vi "SPD.HV_Bias SubTest.vi"(0 "SPD.Stand Ctrl in":T4={"spdDeviceSession"={"spdRef"=0, "connected"=FALSE, "spdName"="", "specification"={"diod case"=enum."default", "type"=enum."Unknown", "frequency"=enum."Unknown"}, "hidSPD.Controller"={"TSet"=0.0, "HV_bias"=0.0, "DDS_stb_code"=0}, "hidSPD.Sturtup Values"={"TSet"=0.0, "HV_bias"=0.0, "DDS_stb_code"=0}}, "DevBSession"={"DevBRef"="", "connected"=FALSE}, "FreqCSession"={"FreqCRef"="", "timeout"=0.0, "Gate"=0.0, "connected"=FALSE}, "8164BSession"={"Connection ID"=refnum, "Connected"=FALSE, "Info"="", "Slots Info"=[]}, "LeCroySession"={"LeCroySession"="", "connected"=FALSE}, "Events"={"DCRTest"=refnum, "Stop"=refnum}, "configFile"={"configFile ref"=refnum, "configFile path"=path "", "equipmentFile ref"=refnum}, "SPD.Meas Grid"={"DateTime"="", "DT"=[], "Insensitivity"=[], "Temprature"=[], "Stb_code"=[], "HV_Bias"=[]}, "SPD.Queues"={"state queue"=refnum}, "Console"=refnum} {"spdDeviceSession"."hidSPD.Sturtup Values"."HV_bias" format="%#_6p, V"; "spdDeviceSession"."hidSPD.Sturtup Values"."TSet" format="%#_6p, DegC"; "spdDeviceSession"."hidSPD.Controller"."HV_bias" format="%#_6p, V"; "spdDeviceSession"."hidSPD.Controller"."TSet" format="%#_6p, DegC"}, 5 "SPD.HV_bias Test Limits":T1, 11 "Error In":errorcluster, 12 "Progress":refnum<vi>, 13 "Graph":refnum<vi>) -> (4 "SPD.Stand Ctrl out":T4={"spdDeviceSession"={"spdRef"=0, "connected"=FALSE, "spdName"="", "specification"={"diod case"=enum."default", "type"=enum."Unknown", "frequency"=enum."Unknown"}, "hidSPD.Controller"={"TSet"=0.0, "HV_bias"=0.0, "DDS_stb_code"=0}, "hidSPD.Sturtup Values"={"TSet"=0.0, "HV_bias"=0.0, "DDS_stb_code"=0}}, "DevBSession"={"DevBRef"="", "connected"=FALSE}, "FreqCSession"={"FreqCRef"="", "timeout"=0.0, "Gate"=0.0, "connected"=FALSE}, "8164BSession"={"Connection ID"=refnum, "Connected"=FALSE, "Info"="", "Slots Info"=[]}, "LeCroySession"={"LeCroySession"="", "connected"=FALSE}, "Events"={"DCRTest"=refnum, "Stop"=refnum}, "configFile"={"configFile ref"=refnum, "configFile path"=path "", "equipmentFile ref"=refnum}, "SPD.Meas Grid"={"DateTime"="", "DT"=[], "Insensitivity"=[], "Temprature"=[], "Stb_code"=[], "HV_Bias"=[]}, "SPD.Queues"={"state queue"=refnum}, "Console"=refnum} {"spdDeviceSession"."hidSPD.Sturtup Values"."HV_bias" format="%#_6p, V"; "spdDeviceSession"."hidSPD.Sturtup Values"."TSet" format="%#_6p, DegC"; "spdDeviceSession"."hidSPD.Controller"."HV_bias" format="%#_6p, V"; "spdDeviceSession"."hidSPD.Controller"."TSet" format="%#_6p, DegC"}, 6 "last HV_bias":dbl, 8 "Clicks Count":dbl, 10 "result":bool, 15 "Error Out":errorcluster)   [LabVIEW 2018]
uses:
  typedefs/SPD.Stand Ctrl.ctl
  Instruments/SPD HID Interface/hidSPDLibForLabView/LibVIs/hidSPD Controls/hidSPD Device Session.ctl
  Instruments/SPD HID Interface/hidSPDLibForLabView/LibVIs/hidSPD Controls/hidSPD.SPD specification.ctl
  Instruments/SPD HID Interface/hidSPDLibForLabView/LibVIs/hidSPD Controls/hidSPD SPD Diod Case.ctl
  Instruments/SPD HID Interface/hidSPDLibForLabView/LibVIs/hidSPD Controls/hidSPD SPD Type.ctl
  Instruments/SPD HID Interface/hidSPDLibForLabView/LibVIs/hidSPD Controls/hidSPD.STB Frequency.ctl
  Instruments/SPD HID Interface/hidSPDLibForLabView/LibVIs/hidSPD Controls/hidSPD Controller.ctl
  Instruments/KC705 DevBoard/typedefs/DevB.Session.ctl
  Instruments/KeySight 53230A/typedefs/FreqC.Session.ctl
  Instruments/KeySight 8164B/KeySight 8164B LAN InstrLib/typedefs/KeySight 8164B control.ctl
  Instruments/LeCroy SDA830/typedefs/LeCroy.Session.ctl
  typedefs/SPD.Events.ctl
  ConfigFile/SPD.Config File ctrl.ctl
  <vilib>/Utility/config.llb/Config Data RefNum.ctl
  typedefs/SPD.Meas Grid.ctl
  typedefs/SPD.Queues.ctl
  typedefs/SPD.Stand state.ctl
  SPD.HV_Bias Test Limits.vi
  SubVIs/Min_Max.ctl
  SubVIs/comparison mode.ctl
  Instruments/SPD HID Interface/hidSPDLibForLabView/LibVIs/hidSPD Controls/hidSPD Controller Setup Report.ctl
  <vilib>/Analysis/1siggen.llb/Ramp Pattern by Delta.vi
  Instruments/SPD HID Interface/hidSPDLibForLabView/LibVIs/hidSPD Write Report/hidSPD Setup Controller.vi
  Instruments/SPD HID Interface/hidSPDLibForLabView/hidSPDLibForLabView.lvlib
  <vilib>/Analysis/NI_AALBase.lvlib
  Instruments/KeySight 8164B/KeySight 8164B LAN InstrLib.lvlib
  <vilib>/Utility/config.llb/NI_LVConfig.lvlib
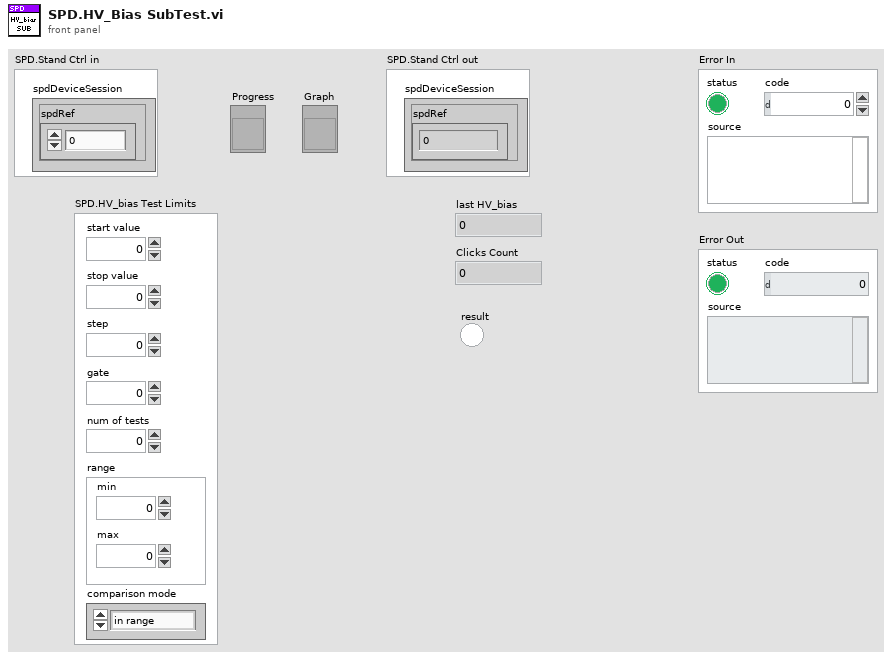
[diagram p1: front panel]
types:
  T1 = typedef "SPD.HV_Bias Test Limits.vi" = cluster{"start value":dbl, "stop value":dbl, "step":dbl, "gate":dbl, "num of tests":dbl, "range":T2, "comparison mode":T3}
  T2 = typedef "Min_Max.ctl" = cluster{"min":dbl, "max":dbl}
  T3 = typedef "comparison mode.ctl" = enum16{"in range", "bigger then min", "bigger then max", "less then min", "less then max"}
  T4 = typedef "SPD.Stand Ctrl.ctl" = cluster{"spdDeviceSession":T5, "DevBSession":T11, "FreqCSession":T12, "8164BSession":T13, "LeCroySession":T14, "Events":T15, "configFile":T16, "SPD.Meas Grid":T18, "SPD.Queues":T19, "Console":refnum<vi>}
  T5 = typedef "hidSPDLibForLabView.lvlib/hidSPD Device Session.ctl" = cluster{"spdRef":u64, "connected":bool, "spdName":string, "specification":T6, "hidSPD.Controller":T10, "hidSPD.Sturtup Values":T10}
  T6 = typedef "hidSPDLibForLabView.lvlib/hidSPD.SPD specification.ctl" = cluster{"diod case":T7, "type":T8, "frequency":T9}
  T7 = typedef "hidSPDLibForLabView.lvlib/hidSPD SPD Diod Case.ctl" = enum16{"Unknown", "default", "butterfly"}
  T8 = typedef "hidSPDLibForLabView.lvlib/hidSPD SPD Type.ctl" = enum16{"Unknown", "Free Run", "Gate"}
  T9 = typedef "hidSPDLibForLabView.lvlib/hidSPD.STB Frequency.ctl" = enum16{"Unknown", "312", "1250"}
  T10 = typedef "hidSPDLibForLabView.lvlib/hidSPD Controller.ctl" = cluster{"TSet":sgl, "HV_bias":sgl, "DDS_stb_code":u16}
  T11 = typedef "DevB.Session.ctl" = cluster{"DevBRef":refnum<visa-resource-name>, "connected":bool}
  T12 = typedef "FreqC.Session.ctl" = cluster{"FreqCRef":refnum<visa-resource-name>, "timeout":dbl, "Gate":dbl, "connected":bool}
  T13 = typedef "KeySight 8164B LAN InstrLib.lvlib/KeySight 8164B control.ctl" = cluster{"Connection ID":refnum<k5>, "Connected":bool, "Info":string, "Slots Info":string[]}
  T14 = typedef "LeCroy.Session.ctl" = cluster{"LeCroySession":refnum<visa-resource-name>, "connected":bool}
  T15 = typedef "SPD.Events.ctl" = cluster{"DCRTest":refnum<user-event>, "Stop":refnum<user-event>}
  T16 = typedef "SPD.Config File ctrl.ctl" = cluster{"configFile ref":T17, "configFile path":path, "equipmentFile ref":T17}
  T17 = typedef "NI_LVConfig.lvlib/Config Data RefNum.ctl" = refnum<k1>
  T18 = typedef "SPD.Meas Grid.ctl" = cluster{"DateTime":string, "DT":dbl[], "Insensitivity":dbl[], "Temprature":dbl[], "Stb_code":dbl[], "HV_Bias":dbl[][][][]}
  T19 = typedef "SPD.Queues.ctl" = cluster{"state queue":refnum<queue>}
  T20 = typedef "hidSPDLibForLabView.lvlib/hidSPD Controller Setup Report.ctl" = cluster{"TSet":sgl, "HV_bias":sgl, "DDS_stb_code":u16, "SPD_reset":u16, "MCU_reset":u16}
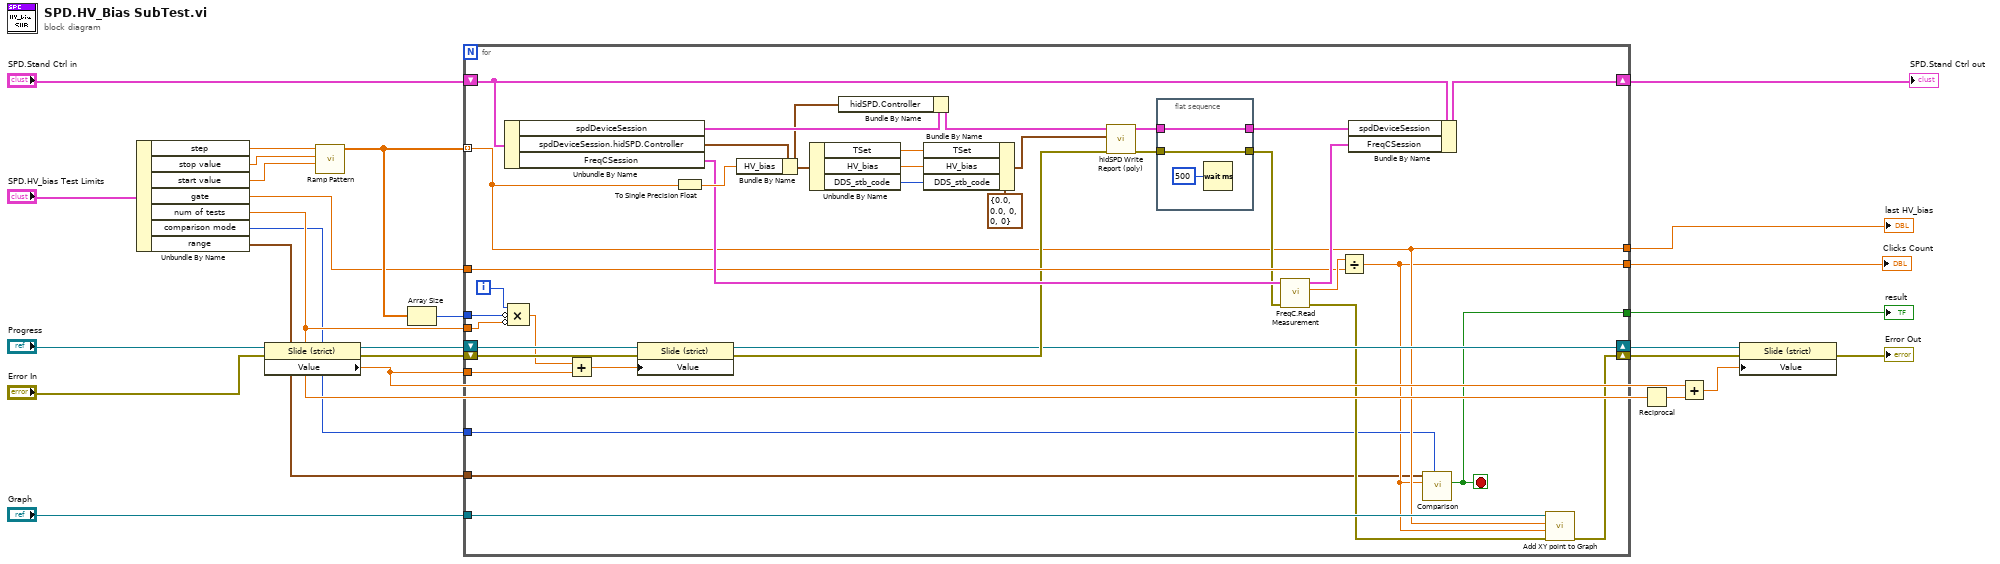
[diagram p0: block diagram]
diagram:
  n1 = Unbundle By Name("SPD.HV_bias Test Limits") -> ("step"=w7:dbl, "stop value"=w6:dbl, "start value"=w5:dbl, "gate"=w4:dbl, "num of tests"=w3:dbl, "comparison mode"=w2:T3, "range"=w1:T2)
  n2 = property class="Slide (strict)"(reference="Progress", error in="Error In") -> (reference out=w21:refnum<vi>, error out=w19:errorcluster, "Value"=w12:dbl)
  n3 = call-poly <vilib>:"Ramp Pattern.vi"("start"=w5, "end"=w6, "delta"=w7) -> ("Ramp Pattern"=w9:dbl[])  [unwired: 6 in, 2 out]
  n4 = Array Size(array=w9) -> (size(s)=w24:i32)
  n5 = for {
    shift-right: [w36] -> w14
    shift-left: w19 -> [w43]
    shift-right: [w53] -> w25
    shift-left: "SPD.Stand Ctrl in" -> [w57]
    tunnel: w9 -> [w38] mode=indexing
    tunnel: w4 -> [w49]
    tunnel: [w35] -> w18
    tunnel: [w38] -> w16
    tunnel: w24 -> [w44]
    shift-right: [w41] -> w15
    shift-left: w21 -> [w40]
    tunnel: "Graph" -> [w39]
    tunnel: [w33] -> w17
    tunnel: w2 -> [w34]
    tunnel: w12 -> [w28]
    tunnel: w1 -> [w31]
    tunnel: w3 -> [w30]
    i -> [w32]
    stop <- w35 stop-if-true
    n6 = Unbundle By Name(w57) -> ("spdDeviceSession"=w64:T5, "spdDeviceSession.hidSPD.Controller"=w62:T10, "FreqCSession"=w51:T12)
    n7 = Compound Arithmetic op=MULTIPLY(w32, invert w44, invert w30) -> (w29:dbl)
    n8 = Add(x=w29, y=w28) -> (x+y=w27:dbl)
    n9 = property class="Slide (strict)"(reference=w40, error in=w43, "Value"=w27) -> (reference out=w41:refnum<vi>, error out=w42:errorcluster)
    n10 = To Single Precision Float(number=w38) -> (single precision float=w52:sgl)
    n11 = Bundle By Name(cluster=w62, "HV_bias"=w52) -> (w55:T10)
    n12 = Unbundle By Name(w55) -> ("TSet"=w61:sgl, "HV_bias"=w60:sgl, "DDS_stb_code"=w59:u16)
    n13 = Bundle By Name(cluster=w64, "hidSPD.Controller"=w55) -> (w56:T5)
    n14 = Bundle By Name(cluster=T20 {"TSet"=0.0, "HV_bias"=0.0, "DDS_stb_code"=0, "SPD_reset"=0, "MCU_reset"=0} ("hidSPD Controller Setup report"), "TSet"=w61, "HV_bias"=w60, "DDS_stb_code"=w59) -> (w58:T20)
    n15 = call-poly "hidSPD Write Report (poly).vi"("error in (no error)"=w42, "hidSPD Controller Setup report"=w58, "spdDevSession in"=w56) -> ("error out"=w47:errorcluster, "spdDevSession out"=w48:T5)  [unwired: 7 in]
    n16 = flat-sequence {
      tunnel: [w67] -> w45
      tunnel: w48 -> [w67]
      tunnel: [w66] -> w46
      tunnel: w47 -> [w66]
      frame #0 {
        n17 = Wait (ms)(milliseconds to wait=u32 500) -> ()  [unwired: 1 out]
      }
    }
    n18 = call "FreqC.Read Measurement.vi"("error In"=w46, "FreqC Session in"=w51) -> ("error out"=w37:errorcluster, "Measurement"=w50:dbl, "FreqC Session out"=w54:T12)  [unwired: 7 in]
    n19 = Divide(x=w50, y=w49) -> (x/y=w33:dbl)
    n20 = Bundle By Name(cluster=w57, "spdDeviceSession"=w45, "FreqCSession"=w54) -> (w53:T4)
    n21 = call "Comparison.vi"("Comparison Mode"=w34, "value"=w33, "minMax"=w31) -> ("result"=w35:bool)  [unwired: 8 in]
    n22 = call "Add XY point to Graph.vi"("error in (no error)"=w37, "Y"=w33, "X"=w38, "Graph in"=w39) -> ("error out"=w36:errorcluster)  [unwired: 6 in, 1 out]
  }
  "SPD.Stand Ctrl out" <- w25
  "result" <- w18
  "Clicks Count" <- w17
  "last HV_bias" <- w16
  n23 = Reciprocal(x=w3) -> (1/x=w11:dbl)
  n24 = Add(x=w12, y=w11) -> (x+y=w10:dbl)
  n25 = property class="Slide (strict)"(reference=w15, error in=w14, "Value"=w10) -> (error out=→"Error Out":errorcluster)  [unwired: 1 out]
